vi "XY Space Adaptation_v1.vi"(9 "deform array":dbl[](array[numeric])=[1.0, 1.0, 1.0, 0.0, 0.0, 0.0, 0.0, 0.0, 0.0], 10 "EyeCenter":dbl[](array[numeric])=[0.0, 10.0], 11 "input (x,y)":dbl[](array[numeric])=[0.0, 10.0]) -> (3 "(x,y) cmd":dbl[](array[numeric]))   [LabVIEW 2010]
doc: "This VI takes in input (x,y) coordinate, compensates for the EyeCenter offset, and output a deformed (x\",y\") using the following formula:\n\n[x',y']' = [x,y]' - EyeCenter;\n[x\",y\"]' = R(theta_z) * diag(x_scaling,y+scaling) * [x',y']' +[x_offset,y_offset]."
uses:
  <vilib>/Analysis/NI_AALBase.lvlib
  <vilib>/Analysis/baseanly.llb/A x Vector.vi
  <vilib>/Analysis/Matrix/NI_Matrix.lvlib
  <vilib>/Analysis/Matrix/Numeric/Conversions/Array To Matrix - RA2.vi
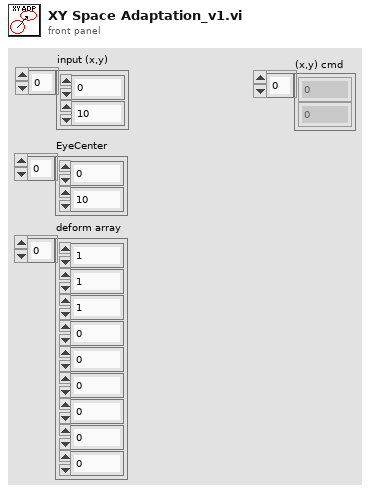
[diagram p1: front panel]
types:
  T1 = typedef "NI_Matrix.lvlib/RealMatrix.ctl" = dbl[][]
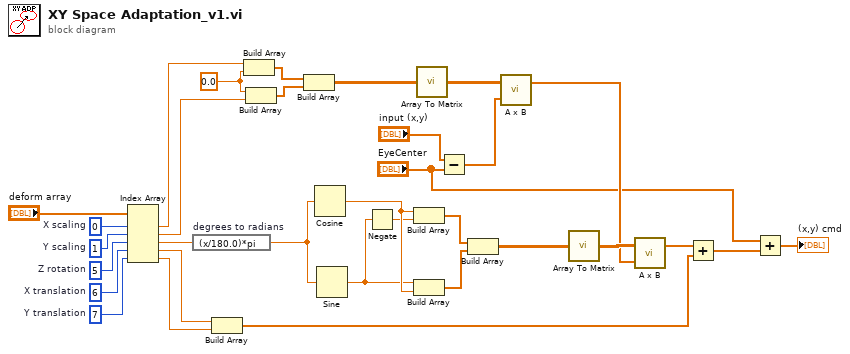
[diagram p0: block diagram]
diagram:
  w18 = 0.0 ("element")
  w26 = 6  # X translation
  w27 = 5  # Z rotation
  w28 = 7  # Y translation
  w29 = 1  # Y scaling
  w30 = 0  # X scaling
  n1 = Index Array(array="deform array", index #1=w30, index #2=w29, index #3=w27, index #4=w26, index #5=w28) -> (element #1=w20:dbl, element #2=w19:dbl, element #3=w25:dbl, element #4=w9:dbl, element #5=w8:dbl)
  n2 = expression code="(x/180.0)*pi" "degrees to radians"(w25) -> (w24:dbl)
  n3 = Build Array(w9, w8) -> (w6:dbl[])
  n4 = Build Array(w20, w18) -> (w16:dbl[])
  n5 = Build Array(w18, w19) -> (w17:dbl[])
  n6 = Build Array(w16, w17) -> (w14:dbl[][])
  n7 = Cosine(x=w24) -> (cos(x)=w23:dbl)
  n8 = Sine(x=w24) -> (sin(x)=w1:dbl)
  n9 = Negate(x=w1) -> (-x=w2:dbl)
  n10 = Build Array(w23, w2) -> (w22:dbl[])
  n11 = Build Array(w1, w23) -> (w21:dbl[])
  n12 = call-poly <vilib>:"Array To Matrix.vi"("Real 2D Array"=w14) -> ("Real Matrix"=w13:T1)
  n13 = Subtract(x="input (x,y)", y="EyeCenter") -> (x-y=w15:dbl[])
  n14 = Build Array(w22, w21) -> (w12:dbl[][])
  n15 = call-poly <vilib>:"A x B.vi"("Vector"=w15, "A"=w13) -> ("A x Vector"=w10:dbl[])  [unwired: 1 out]
  n16 = call-poly <vilib>:"Array To Matrix.vi"("Real 2D Array"=w12) -> ("Real Matrix"=w11:T1)
  n17 = call-poly <vilib>:"A x B.vi"("Vector"=w10, "A"=w11) -> ("A x Vector"=w7:dbl[])  [unwired: 1 out]
  n18 = Add(x=w7, y=w6) -> (x+y=w5:dbl[])
  n19 = Add(x="EyeCenter", y=w5) -> (x+y=→"(x,y) cmd":dbl[])
